vi "Robot Shift (Allen).vi"(10 "speed":dbl, 11 "Move time":dbl) -> (3 "Done":bool)   [LabVIEW 2014]
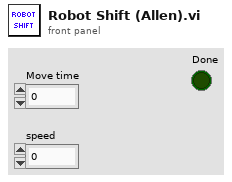
[diagram p1: front panel]
types:
  T1 = typedef "WPI_MotorControlDeviceRef.ctl" = cluster{"DeviceStatus":errorcluster, "Type":T2, "PWM":cluster{"Controller":T3, "PWM Channel":T4, "DeadBand":T5}, "CAN":cluster{"Device Number":u8, "Control Mode":T6, "Semaphore":T7, "Max Vout":dbl, "TalonSRX Control Mode":T8}, "Invert":bool, "TransformRef":T9, "InvTransformRef":T9}
  T2 = typedef "WPI_MotorControlType.ctl" = enum16{"PWM", "CAN", "CANTalonSRX"}
  T3 = typedef "FPGA_TypedefDigitalModule.ctl" = enum16{"Controller 1"}
  T4 = typedef "FPGA_DIOPWMChannel.ctl" = enum8{"PWM 0", "PWM 1", "PWM 2", "PWM 3", "PWM 4", "PWM 5", "PWM 6", "PWM 7", "PWM 8", "PWM 9", "PWM MXP 0", "PWM MXP 1", "PWM MXP 2", "PWM MXP 3", "PWM MXP 4", "PWM MXP 5", "PWM MXP 6", "PWM MXP 7", "PWM MXP 8", "PWM MXP 9", "Invalid"}
  T5 = typedef "WPI_PWMDeadband.ctl" = cluster{"Name":string, "maxPositivePwm":i32, "minPositivePwm":i32, "centerPwm":i32, "maxNegativePwm":i32, "minNegativePwm":i32, "angularRange":u16}
  T6 = typedef "WPI_CANJaguar_ControlMode.ctl" = enum8{"Percent VBus", "Current", "Speed", "Position", "Voltage"}
  T7 = typedef "Semaphore RefNum" = refnum<k1>
  T8 = typedef "WPI_CANTalonSRX_APIControlMode.ctl" = enum8{"Percent VBus", "Speed", "Position", "Slave", "Unchanged / Invalid"}
  T9 = typedef "WPI_PWMTransform_ConPane.ctl" = refnum<vi>
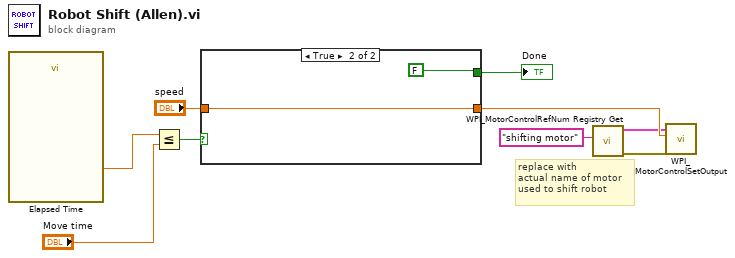
[diagram p0: block diagram]
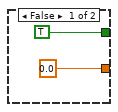
[diagram p2: hidden frame]
diagram:
  # "replace with\nactual name of motor\nused to shift robot"
  n1 = call "Elapsed Time"() -> ("Elapsed Time (s)"=w8:dbl)  [unwired: 12 in, 7 out]
  n2 = Less Or Equal?(x=w8, y="Move time") -> (x <= y?=w6:bool)
  n3 = case shown="True" w6 {
    tunnel: "speed" -> [_ w13]
    tunnel: [0.0 ("speed") w13] -> w7
    tunnel: [TRUE FALSE] -> w1
    frame False {
    }
    frame True {
    }
  }
  "Done" <- w1
  n4 = call <vilib>:"WPI_MotorControlRefNum Registry Get.vi"("refnum name"="shifting motor") -> ("error out"=w3:errorcluster, "MotorControlDevRef"=w2:T1)  [unwired: 9 in]
  n5 = call <vilib>:"WPI_MotorControlSetOutput.vi"("error in (no error)"=w3, "Output"=w7, "MotorControlDevRef"=w2) -> ()  [unwired: 6 in, 3 out]
